vi "Arduino Master Low Level.vi"(0 "Arduino VISA resource index":i32, 1 "Channel Name":string, 2 "VISA resource name":refnum<visa-resource-name>, 3 "Tx msg cluster":T2={"dest"=1, "A/D/C/I"="A", "R/W"="R", "chan"=1, "val (float)"=0.0}) -> (4 "Error":errorcluster, 5 "Value returned":sgl, 6 "Rx checksum ok?":bool, 7 "Tx checksum ok?":bool, 8 "Scan Comments":string="Write Error")   [LabVIEW 2018]
uses:
  ctls_and_globals/Arduino tx msg cluster.ctl
  ctls_and_globals/Arduino Config & resource typedef.ctl
  ctls_and_globals/Arduino Global.vi
panel:
  out "Arduino VISA config & resource":T1={"baud rate (bps)"=276000, "timeout (ms)"=5000, "data bits"=8, "parity"=enum."None", "stop bits (10: 1 bit)"=10, "flow control"=0, "termination char (hex)"=10, "Enable Termination Char"=FALSE, "byte count"=12, "Resource locked?"=FALSE} {"termination char (hex)" format="%02x"; "stop bits (10: 1 bit)" items=["1.0"=10, "1.5"=15, "2.0"=20]; "flow control" items=["None", "XON/XOFF", "RTS/CTS", "XON/XOFF & RTS/CTS", "DTR/DSR", "XON/XOFF & DTR/DSR"]}
  out "Bytes returned":u32
  out "Read buffer (hex)":string
  out "Write buffer (hex)":string
  # "PN custom comms protocol rx / tx msg syntax is 12 bytes: \n'@', src., dest., A/D/C, R/W, chan, val, val ,val, val, rxCHK, txCHK"
  # "Only need to input the following:\ndest, A/D/C, R/W, chan, val, val, val, val\nbyte     str       str    byte            float"
  # "PN 15/07/2013"
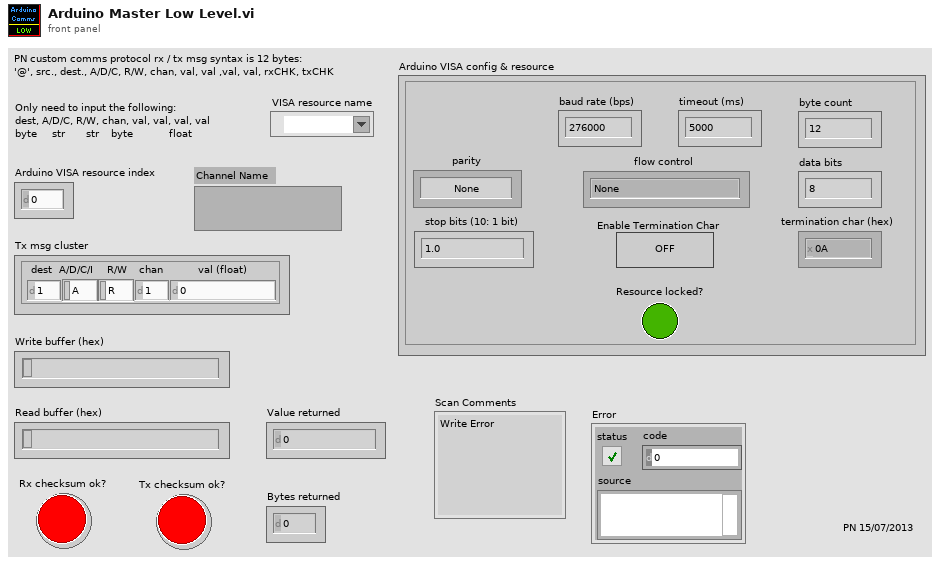
[diagram p1: front panel]
types:
  T1 = typedef "Arduino Config & resource typedef.ctl" = cluster{"baud rate (bps)":u32, "timeout (ms)":u32, "data bits":u16, "parity":enum16{"None", "Odd", "Even", "Mark", "Space"}, "stop bits (10: 1 bit)":u16, "flow control":u16, "termination char (hex)":u8, "Enable Termination Char":bool, "byte count":u32, "Resource locked?":bool}
  T2 = typedef "Arduino tx msg cluster.ctl" = cluster{"dest":u8, "A/D/C/I":string, "R/W":string, "chan":u8, "val (float)":sgl}
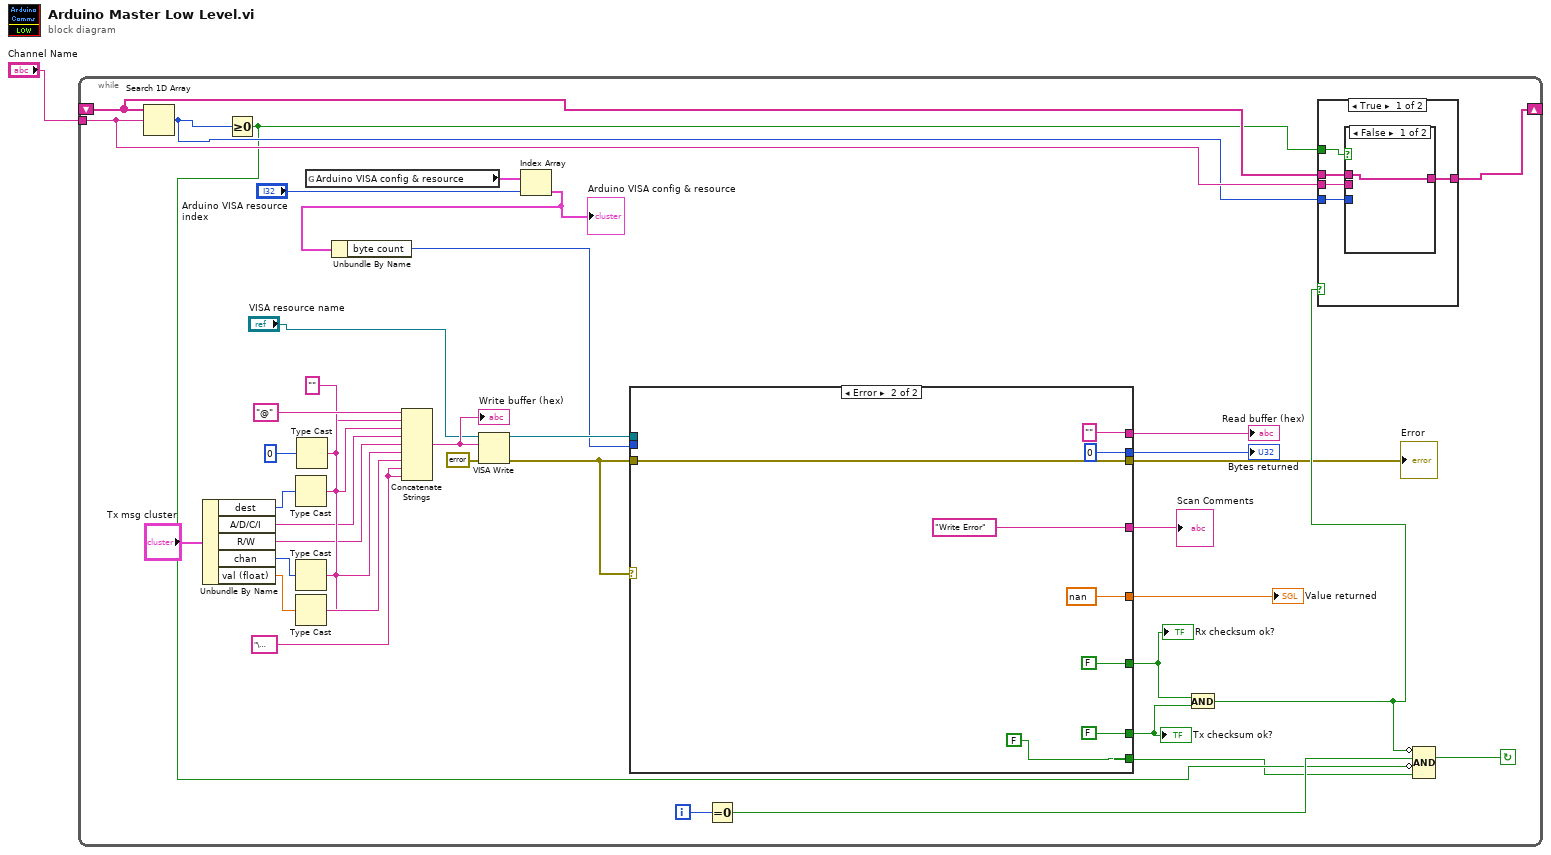
[diagram p0: block diagram]
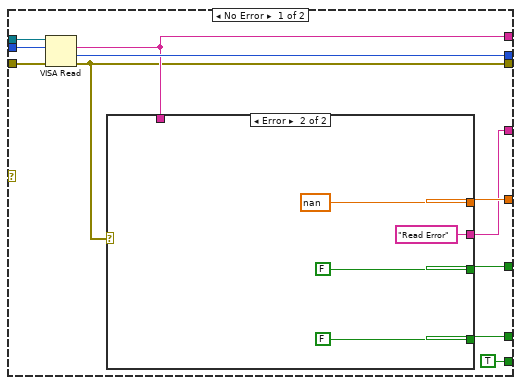
[diagram p2: hidden frame]
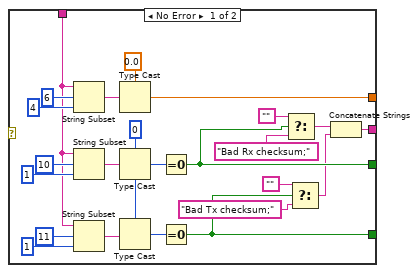
[diagram p3: hidden frame]
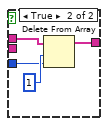
[diagram p4: hidden frame]
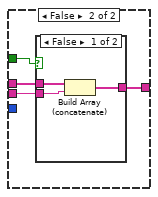
[diagram p5: hidden frame]
diagram:
  n1 = while {
    shift-right: [w16] -> _
    shift-left: _ -> [w14]
    tunnel: "Channel Name" -> [w17]
    i -> [w10]
    stop <- w7 continue-if-true
    w34 = "\u0000"
    w26 = ""
    n2 = Search 1D Array(1D array=w14, element=w17) -> (index of element=w15:i32)  [unwired: 1 in]
    n3 = Unbundle By Name("Tx msg cluster") -> ("dest"=w22:u8, "A/D/C/I"=w21:string, "R/W"=w20:string, "chan"=w19:u8, "val (float)"=w18:sgl)
    n4 = Greater Or Equal To 0?(x=w15) -> (x >= 0?=w8:bool)
    n5 = Type Cast(type=w26, x=w22) -> (*(type *) &x=w37:string)
    n6 = Type Cast(type=w26, x=w19) -> (*(type *) &x=w36:string)
    n7 = Type Cast(type=w26, x=w18) -> (*(type *) &x=w35:string)
    n8 = Type Cast(type=w26, x=u8 0) -> (*(type *) &x=w25:string)
    n9 = global read "Arduino Global.vi" "Arduino VISA config & resource"() -> (w41:T1[])
    n10 = Concatenate Strings("@", w25, w37, w21, w20, w36, w35, w34, w34) -> (w33:string)
    "Write buffer (hex)" <- w33
    n11 = VISA Write(VISA resource name="VISA resource name", write buffer=w33, error in (no error)=errorcluster {"status"=FALSE, "code"=0, "source"=""}) -> (VISA resource name out=w29:refnum<visa-resource-name>, error out=w5:errorcluster)  [unwired: 1 out]
    n12 = Index Array(array=w41, index="Arduino VISA resource index") -> (element=w31:T1)
    "Arduino VISA config & resource" <- w31
    n13 = Unbundle By Name(w31) -> ("byte count"=w28:u32)
    n14 = case shown="Error" w5 {
      tunnel: w5 -> [w52 w85]
      tunnel: [w51 u32 0 ("return count")] -> w30
      tunnel: w29 -> [w50 _]
      tunnel: w28 -> [w49 _]
      tunnel: [w48 "" ("read buffer")] -> w27
      tunnel: [w47 sgl nan] -> w24
      tunnel: [w46 FALSE] -> w13
      tunnel: [w45 FALSE] -> w12
      tunnel: [w44 w85] -> w6
      tunnel: [TRUE FALSE] -> w4
      tunnel: [w42 "Write Error"] -> w3
      frame No Error {
        n15 = VISA Read(VISA resource name=w50, byte count=w49, error in (no error)=w52) -> (read buffer=w48:string, return count=w51:u32, error out=w44:errorcluster)  [unwired: 1 out]
        n16 = case shown="Error" w44 {
          tunnel: w48 -> [w65 _]
          tunnel: [w62 sgl nan] -> w47
          tunnel: [w57 FALSE] -> w46
          tunnel: [w59 FALSE] -> w45
          tunnel: [w53 "Read Error"] -> w42
          frame No Error {
            w74 = u8 0 ("offset (0)")
            n17 = String Subset(string=w65, offset (0)=6, length (rest)=4 ("length (rest)")) -> (substring=w68:string)
            n18 = String Subset(string=w65, offset (0)=10, length (rest)=1 ("length (rest)")) -> (substring=w72:string)
            n19 = String Subset(string=w65, offset (0)=11, length (rest)=1 ("length (rest)")) -> (substring=w73:string)
            n20 = Type Cast(type=sgl 0.0, x=w68) -> (*(type *) &x=w62:sgl)
            n21 = Type Cast(type=w74, x=w72) -> (*(type *) &x=w75:u8)
            n22 = Type Cast(type=w74, x=w73) -> (*(type *) &x=w76:u8)
            n23 = Equal To 0?(x=w75) -> (x = 0?=w57:bool)
            n24 = Equal To 0?(x=w76) -> (x = 0?=w59:bool)
            n25 = Select(t="", s=w57, f="Bad Rx checksum;") -> (s? t:f=w55:string)
            n26 = Select(t="", s=w59, f="Bad Tx checksum;") -> (s? t:f=w54:string)
            n27 = Concatenate Strings(w55, w54) -> (w53:string)
          }
          frame Error {
          }
        }
      }
      frame Error {
      }
    }
    "Read buffer (hex)" <- w27
    "Rx checksum ok?" <- w13
    "Bytes returned" <- w30
    "Tx checksum ok?" <- w12
    "Value returned" <- w24
    "Error" <- w6
    "Scan Comments" <- w3
    n28 = Equal To 0?(x=w10) -> (x = 0?=w9:bool)
    n29 = And(x=w13, y=w12) -> (x .and. y?=w11:bool)
    n30 = case shown="True" w11 {
      tunnel: w8 -> [w93 w102]
      tunnel: w14 -> [w92 w101]
      tunnel: w17 -> [w91 w100]
      tunnel: [w90 w99] -> w16
      tunnel: w15 -> [w89 _]
      frame True {
        n31 = case shown="False" w93 {
          tunnel: w92 -> [w94 w98]
          tunnel: w91 -> [_ _]
          tunnel: [w94 w96] -> w90
          tunnel: w89 -> [_ w95]
          frame False {
          }
          frame True {
            n32 = Delete From Array(array=w98, length=1, index=w95) -> (array with subset deleted=w96:string[])  [unwired: 1 out]
          }
        }
      }
      frame False {
        n33 = case shown="False" w102 {
          tunnel: w101 -> [w105 w106]
          tunnel: w100 -> [w104 _]
          tunnel: [w103 w106] -> w99
          frame False {
            n34 = Build Array (concatenate)(w105, w104) -> (w103:string[])
          }
          frame True {
          }
        }
      }
    }
    n35 = Compound Arithmetic op=AND(invert w11, w9, invert w8, w4) -> (w7:bool)
  }
